vi "Configure Auto Increment Mode.vi"(8 "error in (no error)":errorcluster, 9 "Auto Increment (1:Timer)":u16(ring)=1 items=["Auto Increment OFF", "Timer Mode", "Counter Mode", "Auto Sequence Mode"], 10 "Trigger Value (0000)":i32 format="%04.0f", 11 "VISA resource name":refnum<visa-resource-name>) -> (0 "error out":errorcluster, 3 "VISA resource name out":refnum<visa-resource-name>)   [LabVIEW 2018, in "EFD Ultimus V.lvlib"]
doc: "This VI changes the Auto Increment Mode to either Timer,Counter or Sequence Mode. This command also updates the lower four digits of the trigger value.\n\nHost Format: AC--SsDdddd\nWhere\ns: Mode Command 1=Timer Mode, 2=Counter Mode, 4=Auto Sequence Mode\ndddd: Trigger Value 0001-9999"
uses:
  EFD Ultimus V.lvlib
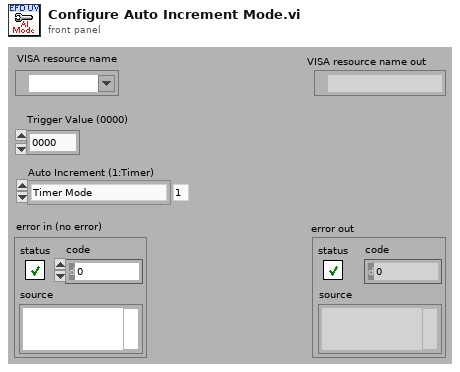
[diagram p1: front panel]
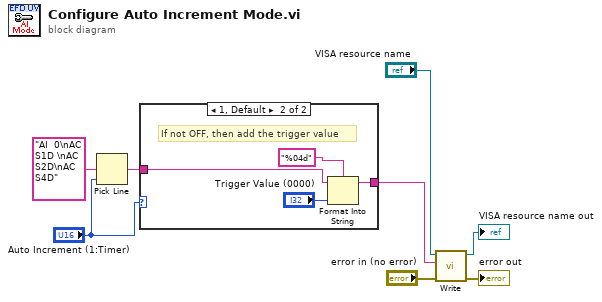
[diagram p0: block diagram]
diagram:
  n1 = Pick Line(multi-line string="AI  0\nAC  S1D \nAC  S2D\nAC  S4D", line index="Auto Increment (1:Timer)") -> (output string=w3:string)  [unwired: 1 in]
  n2 = case shown="1, Default" "Auto Increment (1:Timer)" {
    tunnel: [w9 w10] -> w6
    tunnel: w3 -> [w9 w11]
    frame 0 {
    }
    frame 1, Default {
      # "If not OFF, then add the trigger value"
      n3 = Format Into String(format string="%04d", initial string=w11, "Trigger Value (0000)") -> (resulting string=w10:string)  [unwired: 1 in, 1 out]
    }
  }
  n4 = call "Write.vi"("error in (no error)"="error in (no error)", "Command To Write"=w6, "VISA resource name"="VISA resource name") -> ("error out"=→"error out":errorcluster, "VISA resource name out"=→"VISA resource name out":refnum<visa-resource-name>)  [unwired: 7 out]
